vi "Filter Get Averaging Frame Count.vi"(8 "error in (no error)":errorcluster, 11 "frames":i32) -> (0 "error out":errorcluster, 2 "function return":u32, 3 "frames out":i32)   [LabVIEW 2014, in "atmcd32d.lvlib"]
doc: "unsigned int WINAPI Filter_GetAveragingFrameCount(int * frames);"
uses:
  atmcd32d.lvlib
  atmcd32d.dll
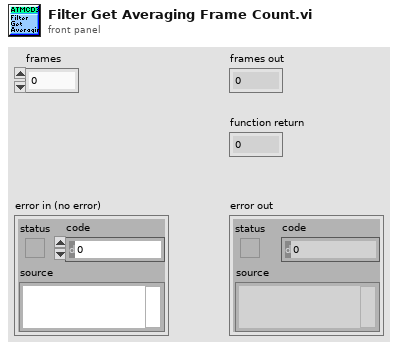
[diagram p1: front panel]
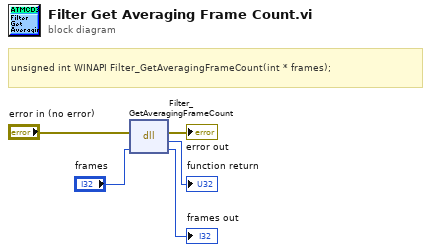
[diagram p0: block diagram]
diagram:
  # "unsigned int WINAPI Filter_GetAveragingFrameCount(int * frames);"
  n1 = dll-call lib="C:/Users/Bakir/Documents/Lambda2-Testing/lib/Andorlib/atmcd32d.*" fn="Filter_GetAveragingFrameCount"(error in="error in (no error)", "frames"="frames") -> (error out=→"error out":errorcluster, →"function return":u32, "frames"=→"frames out":i32)  [unwired: 2 in, 1 out]
